vi "tra25cc_init-config.vi"() -> (3 "conn_xyz_out":T1)   [LabVIEW 2018]
uses:
  D:/Data/Thea/tests/Labview/Scanner_v3_Phy-2019.05.06/src/Stage_xyz/Dll/Newport.CONEXCC.CommandInterface.dll
  Dll/Newport.CONEXCC.CommandInterface.dll
  GLOBAL_VAR.vi
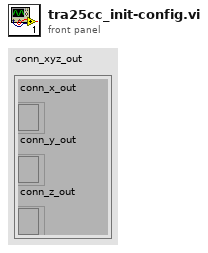
[diagram p1: front panel]
types:
  T1 = cluster{"conn_x_out":refnum<k24>, "conn_y_out":refnum<k24>, "conn_z_out":refnum<k24>}
  T2 = cluster{"COM_X":string, "COM_Y":string, "COM_Z":string}
  T3 = cluster{"conn_x":refnum<k24>, "conn_y":refnum<k24>, "conn_z":refnum<k24>}
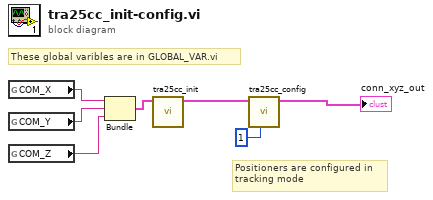
[diagram p0: block diagram]
diagram:
  # "Positioners are configured in\ntracking mode"
  # "These global varibles are in GLOBAL_VAR.vi"
  n1 = global read "GLOBAL_VAR.vi" "COM_X"() -> (w4:string)
  n2 = global read "GLOBAL_VAR.vi" "COM_Y"() -> (w5:string)
  n3 = global read "GLOBAL_VAR.vi" "COM_Z"() -> (w6:string)
  n4 = Bundle("COM_X"=w4, "COM_Y"=w5, "COM_Z"=w6) -> (w1:T2)  [unwired: 1 in]
  n5 = call "tra25cc_init.vi"("com_xyz"=w1) -> ("conn_xyz"=w2:T3)  [unwired: 9 in, 1 out]
  n6 = call "tra25cc_config.vi"("tracking mode"=1, "conn_xyz_in"=w2) -> ("conn_xyz_out"=→"conn_xyz_out":T1)  [unwired: 8 in, 1 out]
